vi "Towerlight.vi"(8 "error in (no error)":errorcluster) -> (0 "error out":errorcluster)   [LabVIEW 2021]
uses:
  Global Variables/FPGA GV.vi
  Global Variables/RT GV.vi
  <vilib>/Utility/error.llb/Error Cluster From Error Code.vi
  <vilib>/rvi/errors/niLvFpgaAdjustHostInterfaceError.vi
  <vilib>/rvi/interface/nirviReadWriteControl/nirviReadWriteControl.xnode
  <vilib>/rvi/interface/Simulation/niFpgaSimulationCallBeginRW.vi
  NiFpgaLv.dll
panel:
  in  "Stop Button in":bool
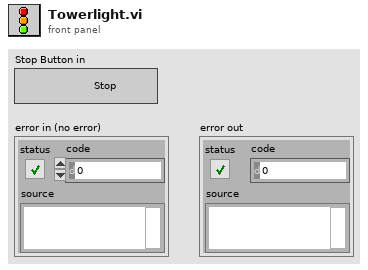
[diagram p1: front panel]
types:
  T1 = cluster{"TL_Red":bool, "TL_Orange":bool, "TL_Green":bool, "TL_Buzzer":bool, "Vaccuum ON":bool, "Vaccuum OFF":bool, "Beckhoff Data":bool, "SOL_Singling":bool, "Bowl Feeder_ ON1":bool, "Buffer 1":bool, "SOL_Pick_Place_Vertical":bool, "SOL_Tube_Feed_Agitatator":bool, "SOL_Tube_Feed_Gating_CYL":bool, "SOL_Insertion _CYL":bool, "SOL_Insertion_Clamp_CYL":bool, "SOL_Cutting_CYL":bool, "SOL_Cutting_Clamp_CYL":bool, "SOL_Insertion_Air_Nozzle":bool, "SOL_Measurement_CYL":bool, "SOL_Pick_Place_Rotary":bool, "SOL_Rejection CYL_1":bool, "SOL_Rejection CYL_2":bool, "SOL_Rejection CYL_3":bool, "SOL_Rejection CYL_4":bool, "Bowl Feeder_ON2":bool, "Linear Feeder 1":bool, "Linear Feeder 2":bool, "Buffer 2":bool, "Buffer 3":bool, "Buffer 4":bool, "Buffer 5":bool, "Buffer 6":bool}
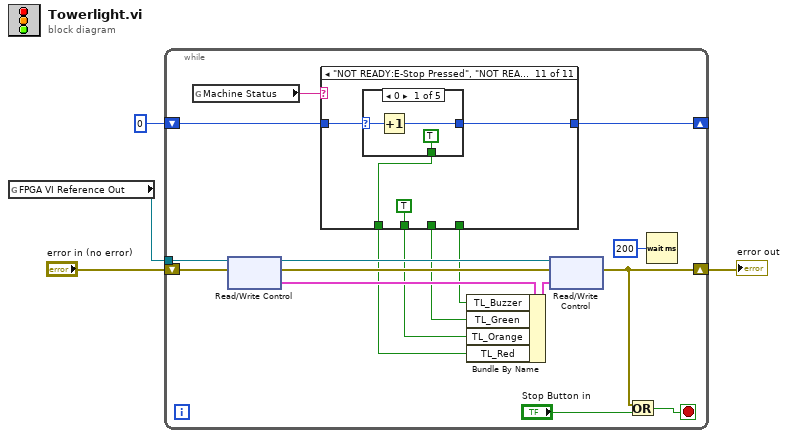
[diagram p0: block diagram]
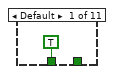
[diagram p2: hidden frame]
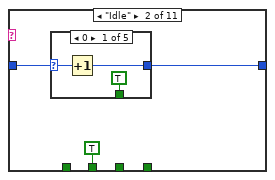
[diagram p3: hidden frame]
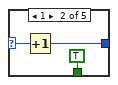
[diagram p4: hidden frame]
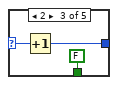
[diagram p5: hidden frame]
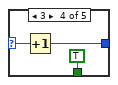
[diagram p6: hidden frame]
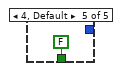
[diagram p7: hidden frame]
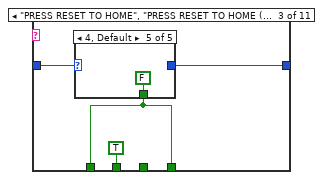
[diagram p8: hidden frame]
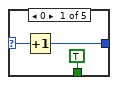
[diagram p9: hidden frame]
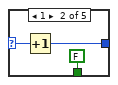
[diagram p10: hidden frame]
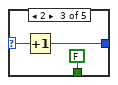
[diagram p11: hidden frame]
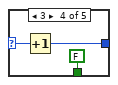
[diagram p12: hidden frame]
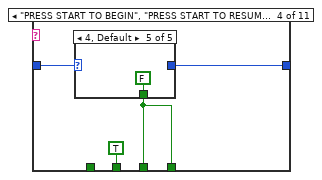
[diagram p13: hidden frame]
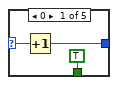
[diagram p14: hidden frame]
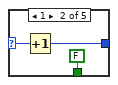
[diagram p15: hidden frame]
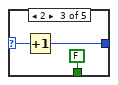
[diagram p16: hidden frame]
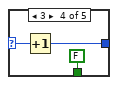
[diagram p17: hidden frame]
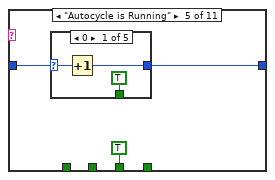
[diagram p18: hidden frame]
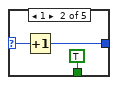
[diagram p19: hidden frame]
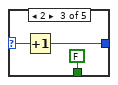
[diagram p20: hidden frame]
diagram:
  n1 = global read "FPGA GV.vi" "FPGA VI Reference Out"() -> (w1:refnum<k20>)
  n2 = while {
    shift-right: [w18] -> w2
    shift-left: "error in (no error)" -> [w14]
    tunnel: w1 -> [w15]
    shift-right: [w16] -> _
    shift-left: 0 -> [w17]
    stop <- w20 stop-if-true
    n3 = global read "RT GV.vi" "Machine Status"() -> (w5:string)
    n4 = xnode "Read/Write Control"("FPGA VI Reference In"=w15, "error in"=w14) -> ("FPGA VI Reference Out"=w13:refnum<k20>, "error out"=w12:errorcluster, "DO 1"=w11:T1)
    n5 = case shown="\"NOT READY:E-Stop Pressed\", \"NOT READY:Front Door is Open\", \"NOT READY:Machine Power\", \"NOT READY:Pneumatic Air\", \"NOT READY:Rear Door(s) are Open\"" w5 {
      tunnel: [_ _ w39 w56 _ _ _ _ _ w156 _] -> w6
      tunnel: [_ _ _ w56 TRUE TRUE w106 w122 _ TRUE _] -> w7
      tunnel: [_ TRUE TRUE TRUE _ w89 _ TRUE w139 _ TRUE] -> w8
      tunnel: [TRUE _ w39 _ _ _ _ _ _ _ w172] -> w9
      tunnel: w17 -> [_ w25 w42 w59 w75 w92 w108 w124 w141 w158 w175]
      tunnel: [_ w24 w41 w58 w74 w91 w107 w123 w140 w157 w174] -> w16
      frame Default {
      }
      frame "Idle" {
        n6 = case shown="0" w25 {
          selector: w25 -> [w28 w31 w34 w37 _]
          tunnel: [w27 w30 w33 w36 _] -> w24
          tunnel: [TRUE TRUE FALSE TRUE FALSE] -> _
          frame 0 {
            n7 = Increment(x=w28) -> (x+1=w27:i32)
          }
          frame 1 {
            n8 = Increment(x=w31) -> (x+1=w30:i32)
          }
          frame 2 {
            n9 = Increment(x=w34) -> (x+1=w33:i32)
          }
          frame 3 {
            n10 = Increment(x=w37) -> (x+1=w36:i32)
          }
          frame 4, Default {
          }
        }
      }
      frame "PRESS RESET TO HOME", "PRESS RESET TO HOME (CHECK ERROR BELOW)" {
        n11 = case shown="4, Default" w42 {
          selector: w42 -> [w45 w48 w51 w54 _]
          tunnel: [w44 w47 w50 w53 _] -> w41
          tunnel: [TRUE FALSE FALSE FALSE FALSE] -> w39
          frame 0 {
            n12 = Increment(x=w45) -> (x+1=w44:i32)
          }
          frame 1 {
            n13 = Increment(x=w48) -> (x+1=w47:i32)
          }
          frame 2 {
            n14 = Increment(x=w51) -> (x+1=w50:i32)
          }
          frame 3 {
            n15 = Increment(x=w54) -> (x+1=w53:i32)
          }
          frame 4, Default {
          }
        }
      }
      frame "PRESS START TO BEGIN", "PRESS START TO RESUME (CHECK ERROR BELOW)" {
        n16 = case shown="4, Default" w59 {
          selector: w59 -> [w62 w65 w68 w71 _]
          tunnel: [w61 w64 w67 w70 _] -> w58
          tunnel: [TRUE FALSE FALSE FALSE FALSE] -> w56
          frame 0 {
            n17 = Increment(x=w62) -> (x+1=w61:i32)
          }
          frame 1 {
            n18 = Increment(x=w65) -> (x+1=w64:i32)
          }
          frame 2 {
            n19 = Increment(x=w68) -> (x+1=w67:i32)
          }
          frame 3 {
            n20 = Increment(x=w71) -> (x+1=w70:i32)
          }
          frame 4, Default {
          }
        }
      }
      frame "Autocycle is Running" {
        n21 = case shown="0" w75 {
          selector: w75 -> [w78 w81 w84 w87 _]
          tunnel: [w77 w80 w83 w86 _] -> w74
          tunnel: [TRUE TRUE FALSE TRUE FALSE] -> _
          frame 0 {
            n22 = Increment(x=w78) -> (x+1=w77:i32)
          }
          frame 1 {
            n23 = Increment(x=w81) -> (x+1=w80:i32)
          }
          frame 2 {
            n24 = Increment(x=w84) -> (x+1=w83:i32)
          }
          frame 3 {
            n25 = Increment(x=w87) -> (x+1=w86:i32)
          }
          frame 4, Default {
          }
        }
      }
      frame "Autocycle is Running (TUBES LOW)" {
        n26 = case shown="0" w92 {
          selector: w92 -> [w95 w98 w101 w104 _]
          tunnel: [w94 w97 w100 w103 _] -> w91
          tunnel: [TRUE FALSE TRUE FALSE TRUE] -> w89
          frame 0 {
            n27 = Increment(x=w95) -> (x+1=w94:i32)
          }
          frame 1 {
            n28 = Increment(x=w98) -> (x+1=w97:i32)
          }
          frame 2 {
            n29 = Increment(x=w101) -> (x+1=w100:i32)
          }
          frame 3 {
            n30 = Increment(x=w104) -> (x+1=w103:i32)
          }
          frame 4, Default {
          }
        }
      }
      frame "Autocycle:Ending Production" {
        n31 = case shown="0" w108 {
          selector: w108 -> [w111 w114 w117 w120 _]
          tunnel: [w110 w113 w116 w119 _] -> w107
          tunnel: [TRUE TRUE TRUE FALSE FALSE] -> w106
          frame 0 {
            n32 = Increment(x=w111) -> (x+1=w110:i32)
          }
          frame 1 {
            n33 = Increment(x=w114) -> (x+1=w113:i32)
          }
          frame 2 {
            n34 = Increment(x=w117) -> (x+1=w116:i32)
          }
          frame 3 {
            n35 = Increment(x=w120) -> (x+1=w119:i32)
          }
          frame 4, Default {
          }
        }
      }
      frame "Autocycle:Homing" {
        n36 = case shown="2" w124 {
          selector: w124 -> [w128 w131 w134 w137 _]
          tunnel: [w127 w130 w133 w136 _] -> w123
          tunnel: [TRUE FALSE TRUE FALSE TRUE] -> w122
          frame 0 {
            n37 = Increment(x=w128) -> (x+1=w127:i32)
          }
          frame 1 {
            n38 = Increment(x=w131) -> (x+1=w130:i32)
          }
          frame 2 {
            n39 = Increment(x=w134) -> (x+1=w133:i32)
          }
          frame 3 {
            n40 = Increment(x=w137) -> (x+1=w136:i32)
          }
          frame 4, Default {
          }
        }
      }
      frame "Maintenance" {
        n41 = case shown="0" w141 {
          selector: w141 -> [w144 w147 w150 w153 _]
          tunnel: [w143 w146 w149 w152 _] -> w140
          tunnel: [TRUE TRUE TRUE FALSE FALSE] -> w139
          frame 0 {
            n42 = Increment(x=w144) -> (x+1=w143:i32)
          }
          frame 1 {
            n43 = Increment(x=w147) -> (x+1=w146:i32)
          }
          frame 2 {
            n44 = Increment(x=w150) -> (x+1=w149:i32)
          }
          frame 3 {
            n45 = Increment(x=w153) -> (x+1=w152:i32)
          }
          frame 4, Default {
          }
        }
      }
      frame "Autocycle:Clear Rejects" {
        n46 = case shown="0" w158 {
          selector: w158 -> [w161 w164 w167 w170 _]
          tunnel: [w160 w163 w166 w169 _] -> w157
          tunnel: [TRUE TRUE TRUE TRUE FALSE] -> w156
          frame 0 {
            n47 = Increment(x=w161) -> (x+1=w160:i32)
          }
          frame 1 {
            n48 = Increment(x=w164) -> (x+1=w163:i32)
          }
          frame 2 {
            n49 = Increment(x=w167) -> (x+1=w166:i32)
          }
          frame 3 {
            n50 = Increment(x=w170) -> (x+1=w169:i32)
          }
          frame 4, Default {
          }
        }
      }
      frame "NOT READY:E-Stop Pressed", "NOT READY:Front Door is Open", "NOT READY:Machine Power", "NOT READY:Pneumatic Air", "NOT READY:Rear Door(s) are Open" {
        n51 = case shown="0" w175 {
          selector: w175 -> [w178 w181 w184 w187 _]
          tunnel: [w177 w180 w183 w186 _] -> w174
          tunnel: [TRUE TRUE TRUE FALSE FALSE] -> w172
          frame 0 {
            n52 = Increment(x=w178) -> (x+1=w177:i32)
          }
          frame 1 {
            n53 = Increment(x=w181) -> (x+1=w180:i32)
          }
          frame 2 {
            n54 = Increment(x=w184) -> (x+1=w183:i32)
          }
          frame 3 {
            n55 = Increment(x=w187) -> (x+1=w186:i32)
          }
          frame 4, Default {
          }
        }
      }
    }
    n56 = Bundle By Name(cluster=w11, "TL_Buzzer"=w6, "TL_Green"=w7, "TL_Orange"=w8, "TL_Red"=w9) -> (w10:T1)
    n57 = xnode "Read/Write Control"("FPGA VI Reference In"=w13, "error in"=w12, "DO 1"=w10) -> ("error out"=w18:errorcluster)  [unwired: 1 out]
    n58 = Or(x=w18, y="Stop Button in") -> (x .or. y?=w20:bool)
    n59 = Wait (ms)(milliseconds to wait=u32 200) -> ()  [unwired: 1 out]
  }
  "error out" <- w2
